vi "Execute.vi"(6 "QD Text":string, 7 "QD Plugins Dir":path, 8 "error in (no error)":errorcluster, 9 "Shift?":bool, 10 "Focus":enum8{"FP", "BD"}(ring), 11 "VI Refnum":refnum<vi>) -> (0 "error out":errorcluster)   [LabVIEW 2019, in "Script.lvlib"]
doc: "Executes scripts shortcuts defined in the Quick Drop arguments.\n\nHelp: Ctrl-Space + \"?\" + Ctrl-S\n\nCreated by: Ryan Pacini"
uses:
  Script.lvlib
  Definitions.ctl
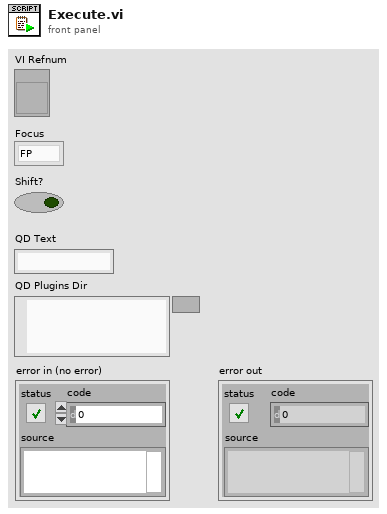
[diagram p1: front panel]
types:
  T1 = typedef "Script.lvlib/Definitions.ctl" = cluster{"plugins":cluster{"vi":path, "desc":string}[], "defaults":cluster{"uid":string, "name":string}[], "shortcuts":cluster{"shortcut":string, "uids":string[]}[], "defaults?":bool}
  T2 = enum16{"open", "replace", "create", "open or create", "replace or create", "replace or create with confirmation"}
  T3 = cluster{"name":string, "default":cluster{"uid":string, "name":string}}
  T4 = cluster{"name":string, "default":cluster{"uid":string, "name":string}}[]
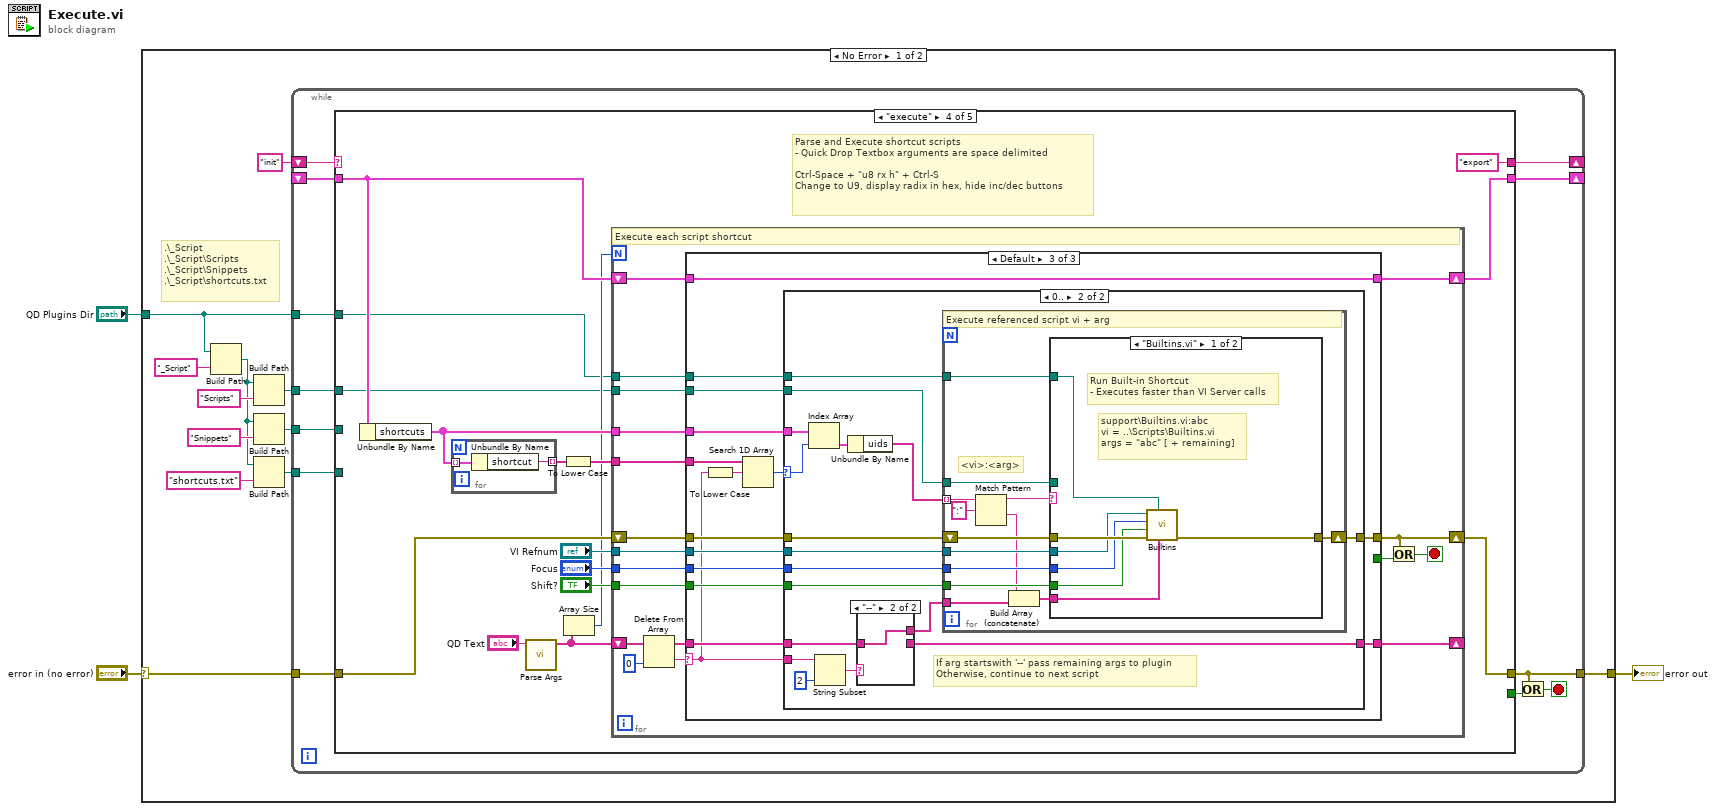
[diagram p0: block diagram]
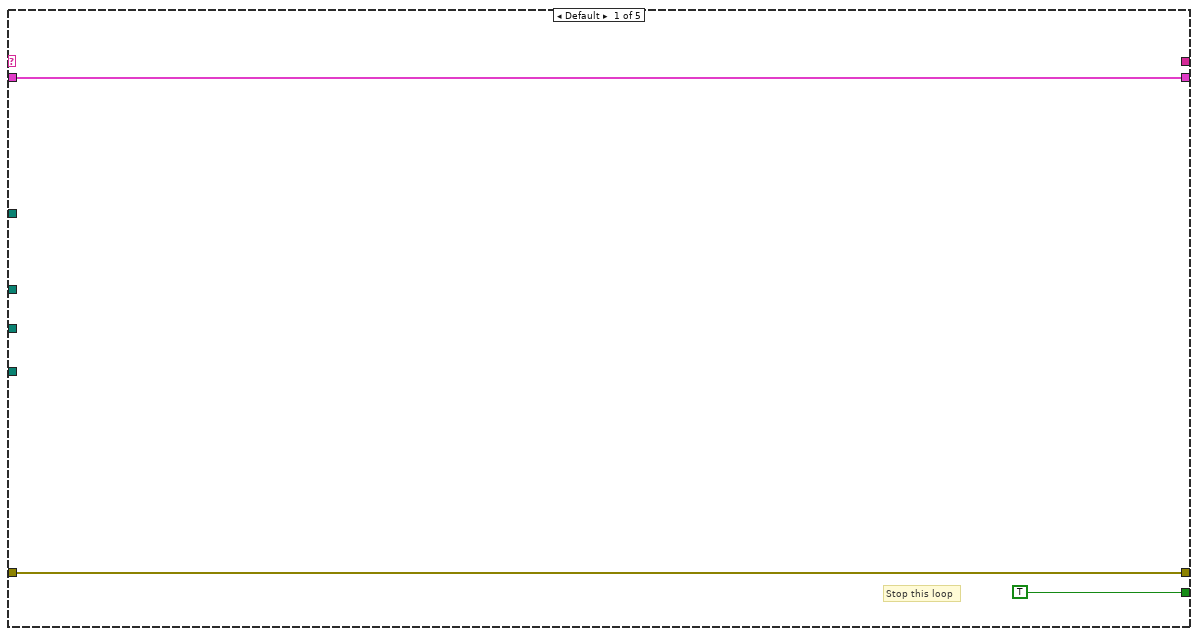
[diagram p2: hidden frame]
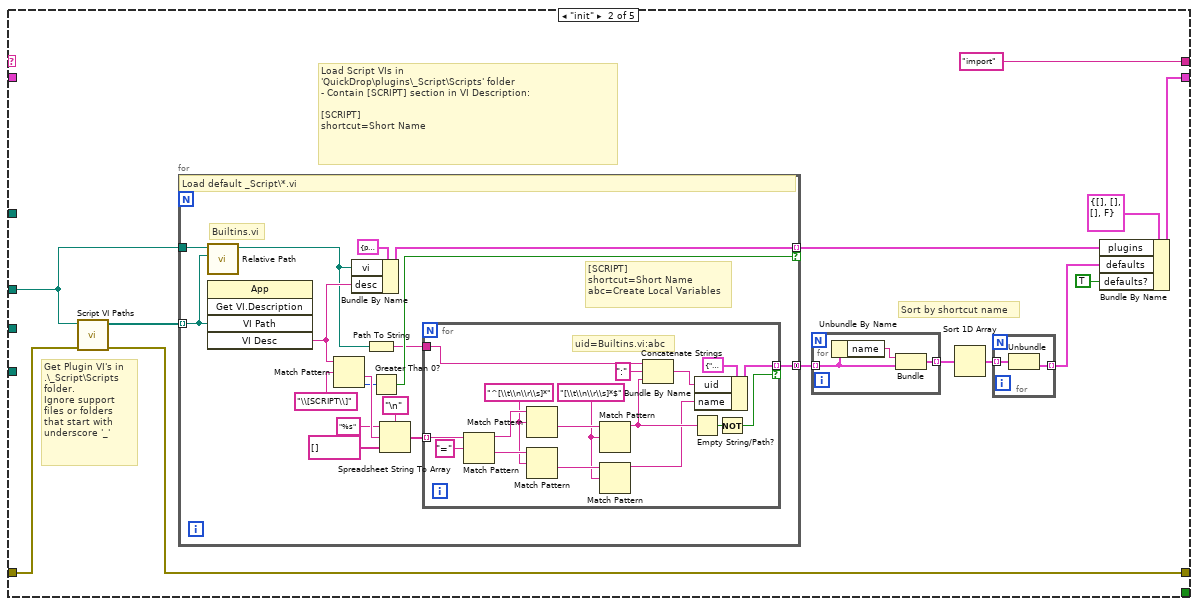
[diagram p3: hidden frame]
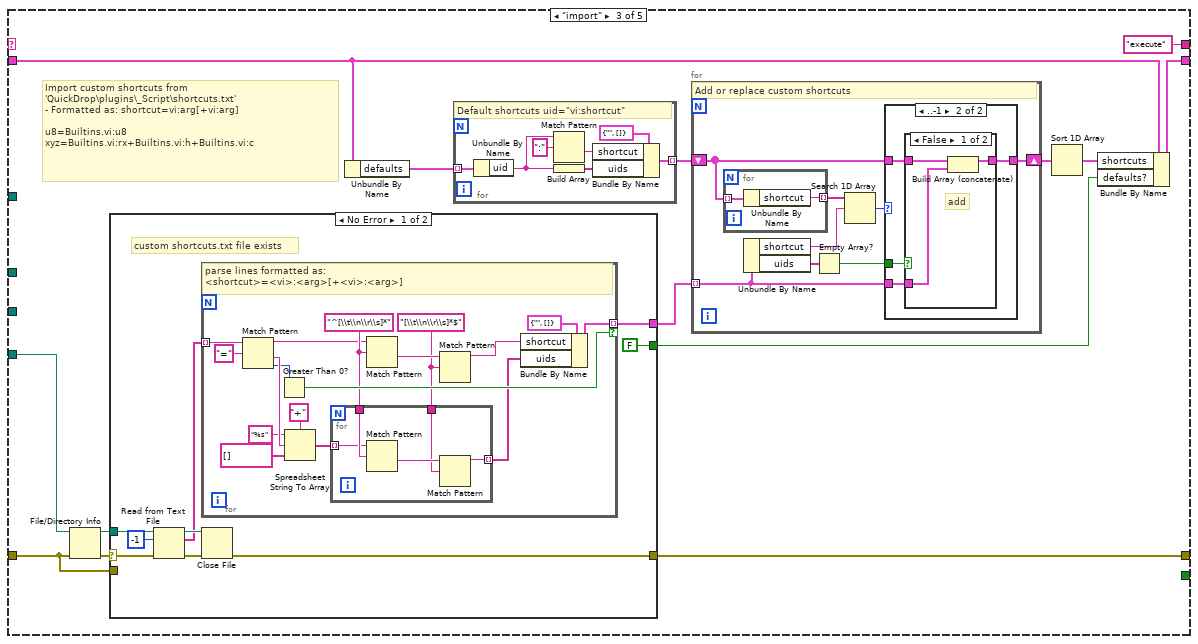
[diagram p4: hidden frame]
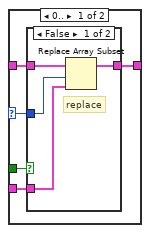
[diagram p5: hidden frame]
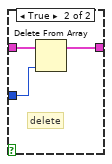
[diagram p6: hidden frame]
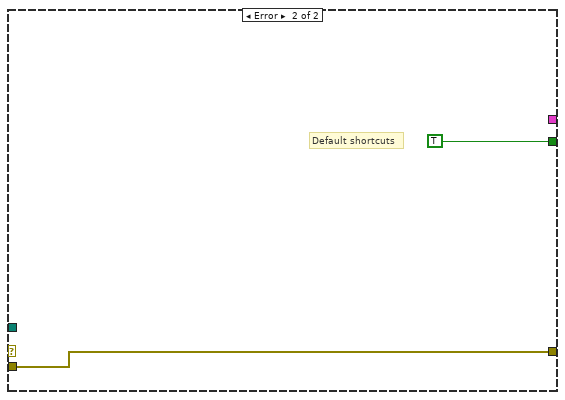
[diagram p8: hidden frame]
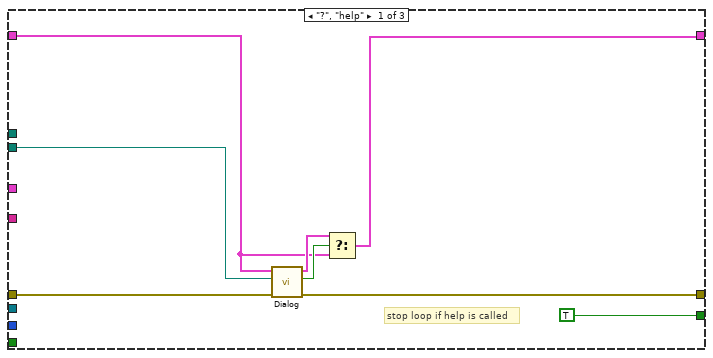
[diagram p9: hidden frame]
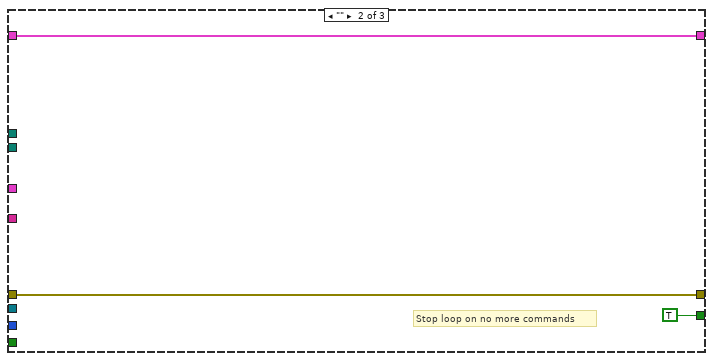
[diagram p10: hidden frame]
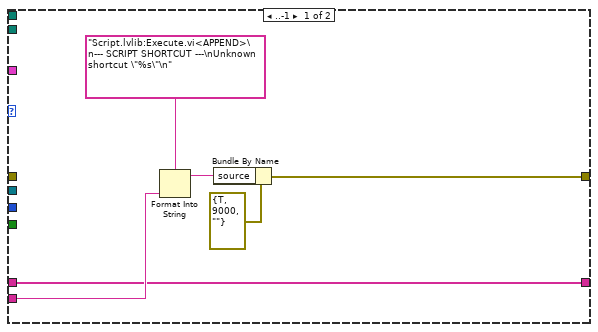
[diagram p11: hidden frame]
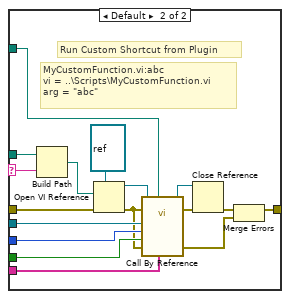
[diagram p13: hidden frame]
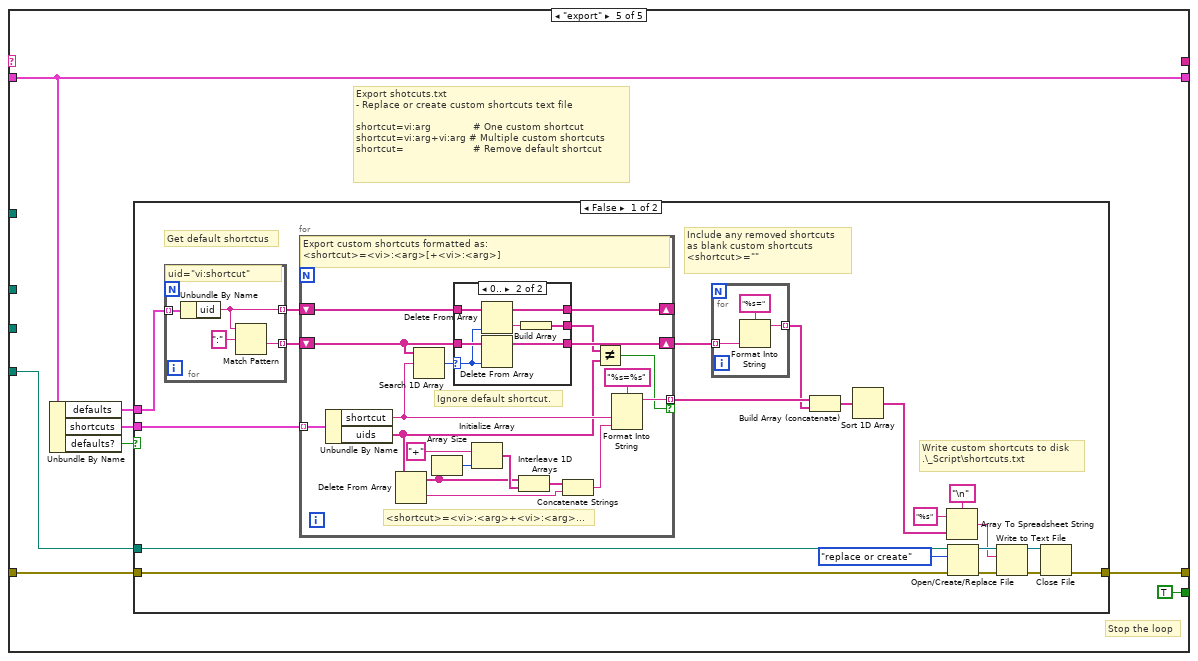
[diagram p14: hidden frame]
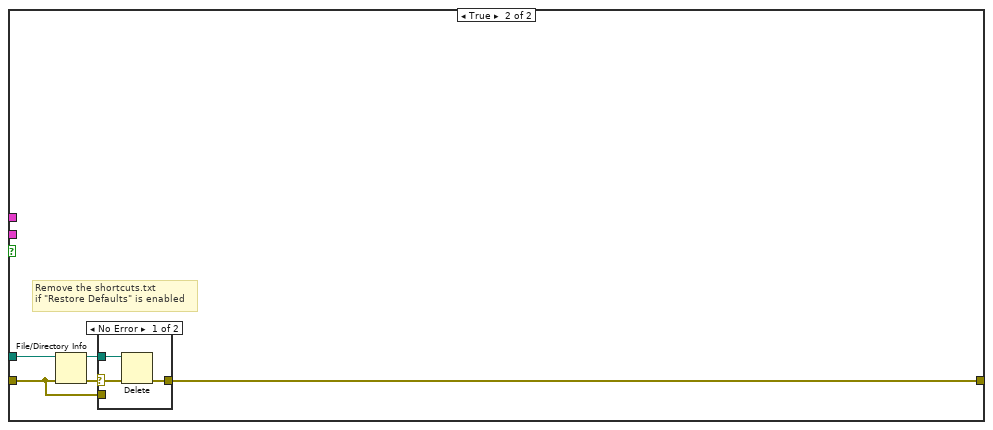
[diagram p16: hidden frame]
diagram:
  n1 = case shown="No Error" "error in (no error)" {
    selector: "error in (no error)" -> [w14 w362]
    tunnel: [w12 w362] -> w2
    tunnel: "QD Plugins Dir" -> [w10 _]
    frame No Error {
      # ".\\_Script\n.\\_Script\\Scripts\n.\\_Script\\Snippets\n.\\_Script\\shortcuts.txt"
      n2 = Build Path(base path=w10, name or relative path="_Script") -> (appended path=w4:path)
      n3 = Build Path(base path=w4, name or relative path="Scripts") -> (appended path=w8:path)
      n4 = Build Path(base path=w4, name or relative path="Snippets") -> (appended path=w5:path)
      n5 = Build Path(base path=w4, name or relative path="shortcuts.txt") -> (appended path=w9:path)
      n6 = while {
        tunnel: w14 -> [w27]
        shift-right: [w25] -> _
        shift-left: "init" -> [w26]
        shift-right: [w24] -> _
        shift-left: _ -> [w23]
        tunnel: [w22] -> w12
        tunnel: w10 -> [w19]
        tunnel: w9 -> [w18]
        tunnel: w8 -> [w17]
        tunnel: w5 -> [w16]
        stop <- w21 stop-if-true
        n7 = case shown="\"execute\"" w26 {
          tunnel: w27 -> [w29 w35 w92 w181 w297]
          tunnel: [_ "import" "execute" "export" _] -> w25
          tunnel: [w30 w42 w90 w175 w294] -> w24
          tunnel: w23 -> [w30 _ w86 w171 w294]
          tunnel: [w29 w34 w95 w177 w296] -> w22
          tunnel: [TRUE _ _ _ TRUE] -> w20
          tunnel: w19 -> [_ _ _ w166 _]
          tunnel: w18 -> [_ _ w91 _ w295]
          tunnel: w17 -> [_ w31 _ w167 _]
          tunnel: w16 -> [_ _ _ _ _]
          frame Default {
            # "Stop this loop"
          }
          frame "init" {
            # "Load Script VIs in \n'QuickDrop\\plugins\\_Script\\Scripts' folder\n- Contain [SCRIPT] section in VI Description:\n\n[SCRIPT]\nshortcut=Short Name"
            # "Get Plugin VI's in \n.\\_Script\\Scripts \nfolder.\nIgnore support \nfiles or folders\nthat start with\nunderscore '_'"
            # "Sort by shortcut name"
            n8 = call "Script VI Paths.vi"("error in (no error)"=w35, "Directory"=w31) -> ("error out"=w34:errorcluster, "VI Paths"=w33:path[])  [unwired: 8 in]
            n9 = for {
              tunnel: w33 -> [w64] mode=indexing
              tunnel: [w63] -> w40 mode=indexing if=w62
              tunnel: w31 -> [w61]
              tunnel: [w60] -> w39 mode=concatenating
              # "Builtins.vi"
              # "[SCRIPT]\nshortcut=Short Name\nabc=Create Local Variables"
              # "Load default _Script\\*.vi"
              n10 = call "Relative Path.vi"("Child"=w64, "Parent"=w61) -> ("Child Relative Path"=w49:path)  [unwired: 9 in]
              n11 = invoke class="App" method="Get VI.Description"("VI Path"=w64) -> ("VI Desc"=w51:string)  [unwired: 4 in, 4 out]
              n12 = Match Pattern(string=w51, regular expression="\\[SCRIPT\\]") -> (after substring=w58:string, offset past match=w53:i32)  [unwired: 1 in, 2 out]
              n13 = Bundle By Name(cluster=cluster{"vi":path, "desc":string} {"vi"=path "", "desc"=""} ("plugin"), "vi"=w49, "desc"=w51) -> (w63:cluster{"vi":path, "desc":string})
              n14 = Path To String(path=w49) -> (string=w50:string)
              n15 = Greater Than 0?(x=w53) -> (x > 0?=w62:bool)
              n16 = Spreadsheet String To Array(delimiter (Tab)="\n", format string="%s", spreadsheet string=w58, array type (2D Dbl)=string[] []) -> (array=w54:string[])
              n17 = for {
                tunnel: w54 -> [w81] mode=indexing
                tunnel: [w66] -> w60 mode=indexing if=w72
                tunnel: w50 -> [w70]
                w74 = "[\\t\\n\\r\\s]*$" ("regular expression")
                w75 = "^[\\t\\n\\r\\s]*" ("regular expression")
                # "uid=Builtins.vi:abc"
                n18 = Match Pattern(string=w81, regular expression="=") -> (before substring=w78:string, after substring=w76:string)  [unwired: 1 in, 2 out]
                n19 = Match Pattern(string=w78, regular expression=w75) -> (after substring=w79:string)  [unwired: 1 in, 3 out]
                n20 = Match Pattern(string=w76, regular expression=w75) -> (after substring=w77:string)  [unwired: 1 in, 3 out]
                n21 = Match Pattern(string=w79, regular expression=w74) -> (before substring=w69:string)  [unwired: 1 in, 3 out]
                n22 = Match Pattern(string=w77, regular expression=w74) -> (before substring=w65:string)  [unwired: 1 in, 3 out]
                n23 = Concatenate Strings(w70, ":" ("string"), w69) -> (w67:string)
                n24 = Empty String/Path?(string/path=w69) -> (empty?=w73:bool)
                n25 = Bundle By Name(cluster=cluster{"uid":string, "name":string} {"uid"="", "name"=""} ("default"), "uid"=w67, "name"=w65) -> (w66:cluster{"uid":string, "name":string})
                n26 = Not(x=w73) -> (.not. x?=w72:bool)
              }
            }
            n27 = for {
              tunnel: w39 -> [w47] mode=indexing
              tunnel: [w46] -> w38 mode=indexing
              n28 = Unbundle By Name(w47) -> ("name"=w48:string)
              n29 = Bundle("name"=w48, "default"=w47) -> (w46:T3)  [unwired: 1 in]
            }
            n30 = Sort 1D Array(array=w38) -> (sorted array=w37:T4)
            n31 = for {
              tunnel: w37 -> [w45] mode=indexing
              tunnel: [w44] -> w36 mode=indexing
              n32 = Unbundle(w45) -> ("default"=w44:cluster{"uid":string, "name":string})  [unwired: 1 out]
            }
            n33 = Bundle By Name(cluster=T1 {"plugins"=[], "defaults"=[], "shortcuts"=[], "defaults?"=FALSE} ("data"), "plugins"=w40, "defaults"=w36, "defaults?"=TRUE) -> (w42:T1)
          }
          frame "import" {
            # "Import custom shortcuts from \n'QuickDrop\\plugins\\_Script\\shortcuts.txt'\n- Formatted as: shortcut=vi:arg[+vi:arg]\n\nu8=Builtins.vi:u8\nxyz=Builtins.vi:rx+Builtins.vi:h+Builtins.vi:c"
            n34 = File/Directory Info(path=w91, error in=w92) -> (path out=w94:path, error out=w93:errorcluster)  [unwired: 5 out]
            n35 = case shown="No Error" w93 {
              selector: w93 -> [w140 _]
              tunnel: [w136 w165] -> w95
              tunnel: w94 -> [w141 _]
              tunnel: w92 -> [_ w165]
              tunnel: [FALSE TRUE] -> w87
              tunnel: [w133 _] -> w82
              frame No Error {
                # "custom shortcuts.txt file exists"
                n36 = Read from Text File(file (use dialog)=w141, count=-1, error in=w140) -> (refnum out=w137:refnum<file>, text=w134:string[], error out=w138:errorcluster)  [unwired: 1 in, 1 out]
                n37 = for {
                  tunnel: w134 -> [w158] mode=indexing
                  tunnel: [w149] -> w133 mode=indexing if=w151
                  w146 = "[\\t\\n\\r\\s]*$" ("regular expression")
                  w147 = "^[\\t\\n\\r\\s]*" ("regular expression")
                  # "parse lines formatted as:\n<shortcut>=<vi>:<arg>[+<vi>:<arg>]"
                  n38 = Match Pattern(string=w158, regular expression="=") -> (before substring=w145:string, after substring=w156:string, offset past match=w152:i32)  [unwired: 1 in, 1 out]
                  n39 = Greater Than 0?(x=w152) -> (x > 0?=w151:bool)
                  n40 = Spreadsheet String To Array(delimiter (Tab)="+", format string="%s", spreadsheet string=w156, array type (2D Dbl)=string[] []) -> (array=w143:string[])
                  n41 = for {
                    tunnel: w147 -> [w162]
                    tunnel: w146 -> [w161]
                    tunnel: w143 -> [w160] mode=indexing
                    tunnel: [w159] -> w142 mode=indexing
                    n42 = Match Pattern(string=w160, regular expression=w162) -> (after substring=w163:string)  [unwired: 1 in, 3 out]
                    n43 = Match Pattern(string=w163, regular expression=w161) -> (before substring=w159:string)  [unwired: 1 in, 3 out]
                  }
                  n44 = Match Pattern(string=w145, regular expression=w147) -> (after substring=w148:string)  [unwired: 1 in, 3 out]
                  n45 = Match Pattern(string=w148, regular expression=w146) -> (before substring=w144:string)  [unwired: 1 in, 3 out]
                  n46 = Bundle By Name(cluster=cluster{"shortcut":string, "uids":string[]} {"shortcut"="", "uids"=[]} ("shortcut"), "shortcut"=w144, "uids"=w142) -> (w149:cluster{"shortcut":string, "uids":string[]})
                }
                n47 = Close File(refnum=w137, error in=w138) -> (error out=w136:errorcluster)  [unwired: 1 out]
              }
              frame Error {
                # "Default shortcuts"
              }
            }
            n48 = Unbundle By Name(w86) -> ("defaults"=w85:cluster{"uid":string, "name":string}[])
            n49 = for {
              tunnel: w85 -> [w131] mode=indexing
              tunnel: [w129] -> w84 mode=indexing
              # "Default shortcuts uid=\"vi:shortcut\""
              n50 = Unbundle By Name(w131) -> ("uid"=w128:string)
              n51 = Match Pattern(string=w128, regular expression=":") -> (after substring=w126:string)  [unwired: 1 in, 3 out]
              n52 = Build Array(w128) -> (w130:string[])
              n53 = Bundle By Name(cluster=cluster{"shortcut":string, "uids":string[]} {"shortcut"="", "uids"=[]} ("shortcut"), "shortcut"=w126, "uids"=w130) -> (w129:cluster{"shortcut":string, "uids":string[]})
            }
            n54 = for {
              shift-right: [w100] -> w83
              shift-left: w84 -> [w103]
              tunnel: w82 -> [w99] mode=indexing
              # "Add or replace custom shortcuts"
              n55 = for {
                tunnel: w103 -> [w125] mode=indexing
                tunnel: [w124] -> w102 mode=indexing
                n56 = Unbundle By Name(w125) -> ("shortcut"=w124:string)
              }
              n57 = Unbundle By Name(w99) -> ("shortcut"=w101:string, "uids"=w97:string[])
              n58 = Empty Array?(array=w97) -> (empty?=w96:bool)
              n59 = Search 1D Array(1D array=w102, element=w101) -> (index of element=w98:i32)  [unwired: 1 in]
              n60 = case shown="..-1" w98 {
                selector: w98 -> [w105 _]
                tunnel: w103 -> [w108 w119]
                tunnel: [w107 w118] -> w100
                tunnel: w99 -> [w106 w117]
                tunnel: w96 -> [w104 w116]
                frame 0.. {
                  n61 = case shown="False" w104 {
                    tunnel: w108 -> [w112 w115]
                    tunnel: [w111 w113] -> w107
                    tunnel: w106 -> [w110 _]
                    tunnel: w105 -> [w109 w114]
                    frame False {
                      # "replace"
                      n62 = Replace Array Subset(array=w112, new element=w110, index=w109) -> (w111:cluster{"shortcut":string, "uids":string[]}[])
                    }
                    frame True {
                      # "delete"
                      n63 = Delete From Array(array=w115, index=w114) -> (array with subset deleted=w113:cluster{"shortcut":string, "uids":string[]}[])  [unwired: 1 in, 1 out]
                    }
                  }
                }
                frame ..-1 {
                  n64 = case shown="False" w116 {
                    tunnel: w119 -> [w122 w123]
                    tunnel: [w121 w123] -> w118
                    tunnel: w117 -> [w120 _]
                    frame False {
                      # "add"
                      n65 = Build Array (concatenate)(w122, w120) -> (w121:cluster{"shortcut":string, "uids":string[]}[])
                    }
                    frame True {
                      # "do not add"
                    }
                  }
                }
              }
            }
            n66 = Sort 1D Array(array=w83) -> (sorted array=w88:cluster{"shortcut":string, "uids":string[]}[])
            n67 = Bundle By Name(cluster=w86, "shortcuts"=w88, "defaults?"=w87) -> (w90:T1)
          }
          frame "execute" {
            # "Parse and Execute shortcut scripts\n- Quick Drop Textbox arguments are space delimited\n\nCtrl-Space + \"u8 rx h\" + Ctrl-S\nChange to U9, display radix in hex, hide inc/dec buttons"
            n68 = Unbundle By Name(w171) -> ("shortcuts"=w172:cluster{"shortcut":string, "uids":string[]}[])
            n69 = for {
              tunnel: w172 -> [w289] mode=indexing
              tunnel: [w288] -> w174 mode=indexing
              n70 = Unbundle By Name(w289) -> ("shortcut"=w288:string)
            }
            n71 = call "Parse Args.vi"("QD Text"="QD Text") -> ("args"=w168:string[])  [unwired: 10 in]
            n72 = To Lower Case(string=w174) -> (all lower case string=w173:string[])
            n73 = Array Size(array=w168) -> (size(s)=w169:i32)
            n74 = for {
              N: w169 -> [_]
              tunnel: w173 -> [w199]
              tunnel: w172 -> [w198]
              tunnel: "VI Refnum" -> [w196]
              tunnel: "Focus" -> [w195]
              tunnel: "Shift?" -> [w194]
              shift-right: [w190] -> w177
              shift-left: w181 -> [w197]
              shift-right: [w193] -> w175
              shift-left: w171 -> [w192]
              tunnel: w167 -> [w191]
              shift-right: [w184] -> _
              shift-left: w168 -> [w188]
              tunnel: w166 -> [w182]
              stop <- w186 stop-if-true
              # "Execute each script shortcut"
              n75 = Delete From Array(array=w188, index=0) -> (deleted portion=w183:string, array with subset deleted=w185:string[])  [unwired: 1 in]
              n76 = case shown="Default" w183 {
                selector: w183 -> [_ _ w213]
                tunnel: w199 -> [_ _ w225]
                tunnel: w198 -> [_ _ w223]
                tunnel: w197 -> [w207 w209 w222]
                tunnel: w196 -> [_ _ w221]
                tunnel: w195 -> [_ _ w220]
                tunnel: w194 -> [_ _ w219]
                tunnel: [w206 w209 w218] -> w190
                tunnel: [w202 w210 w217] -> w193
                tunnel: w192 -> [w203 w210 w217]
                tunnel: w191 -> [w201 _ w216]
                tunnel: [TRUE TRUE _] -> w189
                tunnel: w185 -> [_ _ w215]
                tunnel: [_ _ w214] -> w184
                tunnel: w182 -> [_ _ w211]
                frame "?", "help" {
                  # "stop loop if help is called"
                  n77 = call "Dialog.vi"("error in (no error)"=w207, "Scripts Dir"=w201, "Definitions in"=w203) -> ("error out"=w206:errorcluster, "commit?"=w205:bool, "Definitions out"=w204:T1)  [unwired: 6 in]
                  n78 = Select(t=w204, s=w205, f=w203) -> (s? t:f=w202:T1)
                }
                frame "" {
                  # "Stop loop on no more commands"
                }
                frame Default {
                  n79 = To Lower Case(string=w213) -> (all lower case string=w212:string)
                  n80 = Search 1D Array(1D array=w225, element=w212) -> (index of element=w224:i32)  [unwired: 1 in]
                  n81 = case shown="0.." w224 {
                    selector: w224 -> [_ w248]
                    tunnel: w223 -> [_ w247]
                    tunnel: w222 -> [_ w244]
                    tunnel: w221 -> [_ w243]
                    tunnel: w220 -> [_ w242]
                    tunnel: w219 -> [_ w241]
                    tunnel: [w230 w240] -> w218
                    tunnel: w216 -> [_ w239]
                    tunnel: w213 -> [w229 w237]
                    tunnel: w215 -> [w226 w235]
                    tunnel: [w226 w234] -> w214
                    tunnel: w211 -> [_ w232]
                    frame ..-1 {
                      n82 = Format Into String(format string="Script.lvlib:Execute.vi<APPEND>\n--- SCRIPT SHORTCUT ---\nUnknown shortcut \"%s\"\n" ("source"), w229) -> (resulting string=w227:string)  [unwired: 2 in, 1 out]
                      n83 = Bundle By Name(cluster=errorcluster {"status"=TRUE, "code"=9000, "source"=""} ("error IO"), "source"=w227) -> (w230:errorcluster)
                    }
                    frame 0.. {
                      # "If arg startswith '--' pass remaining args to plugin\nOtherwise, continue to next script"
                      n84 = Index Array(array=w247, index=w248) -> (element=w246:cluster{"shortcut":string, "uids":string[]})
                      n85 = String Subset(string=w237, length (rest)=2 ("length (rest)")) -> (substring=w236:string)  [unwired: 1 in]
                      n86 = Unbundle By Name(w246) -> ("uids"=w245:string[])
                      n87 = case shown="\"--\"" w236 {
                        tunnel: w235 -> [w249 w250]
                        tunnel: [w249 _] -> w234
                        tunnel: [_ w250] -> w233
                        frame Default {
                        }
                        frame "--" {
                        }
                      }
                      n88 = for {
                        tunnel: w245 -> [w257] mode=indexing
                        tunnel: w243 -> [w262]
                        tunnel: w242 -> [w261]
                        tunnel: w241 -> [w260]
                        shift-right: [w259] -> w240
                        shift-left: w244 -> [w263]
                        tunnel: w239 -> [w254]
                        tunnel: w233 -> [w253]
                        tunnel: w232 -> [w251]
                        # "<vi>:<arg>"
                        # "Execute referenced script vi + arg"
                        n89 = Match Pattern(string=w257, regular expression=":") -> (before substring=w255:string, after substring=w258:string)  [unwired: 1 in, 2 out]
                        n90 = Build Array (concatenate)(w258, w253) -> (w252:string[])
                        n91 = case shown="\"Builtins.vi\"" w255 {
                          selector: w255 -> [_ w275]
                          tunnel: w263 -> [w270 w287]
                          tunnel: w262 -> [w269 w284]
                          tunnel: w261 -> [w268 w283]
                          tunnel: w260 -> [w267 w282]
                          tunnel: [w266 w277] -> w259
                          tunnel: w254 -> [_ w274]
                          tunnel: w252 -> [w265 w272]
                          tunnel: w251 -> [w264 w271]
                          frame "Builtins.vi" {
                            # "support\\Builtins.vi:abc\nvi = ..\\Scripts\\Builtins.vi\nargs = \"abc\" [ + remaining]"
                            # "Run Built-in Shortcut\n- Executes faster than VI Server calls"
                            n92 = call "Builtins.vi"("args"=w265, "QD Plugins Dir"=w264, "error in (no error)"=w270, "Shift?"=w267, "Focus"=w268, "VI Refnum"=w269) -> ("error out"=w266:errorcluster)  [unwired: 5 in]
                          }
                          frame Default {
                            # "Run Custom Shortcut from Plugin"
                            # "MyCustomFunction.vi:abc\nvi = ..\\Scripts\\MyCustomFunction.vi\narg = \"abc\""
                            n93 = Build Path(base path=w274, name or relative path=w275) -> (appended path=w273:path)
                            n94 = Open VI Reference(type specifier VI Refnum (for type only)=refnum<vi> refnum, vi path=w273, error in (no error)=w287) -> (vi reference=w285:refnum<vi>, error out=w281:errorcluster)  [unwired: 3 in]
                            n95 = call-by-ref "?"(reference=w285, error in=w281, "args"=w272, "QD Plugins Dir"=w271, 8:"error in (no error)"=w281, "Shift?"=w282, "Focus"=w283, "VI Refnum"=w284) -> (reference out=w279:refnum<vi>, error out=w280:errorcluster, 0:"error out"=w276:errorcluster)  [unwired: 5 in]
                            n96 = Close Reference(reference=w279, error in (no error)=w280) -> (error out=w278:errorcluster)
                            n97 = Merge Errors(w278, w276) -> (w277:errorcluster)
                          }
                        }
                      }
                    }
                  }
                }
              }
              n98 = Or(x=w190, y=w189) -> (x .or. y?=w186:bool)
            }
          }
          frame "export" {
            # "Export shotcuts.txt\n- Replace or create custom shortcuts text file\n\nshortcut=vi:arg              # One custom shortcut\nshortcut=vi:arg+vi:arg # Multiple custom shortcuts\nshortcut=                       # Remove default shortcut"
            # "Stop the loop"
            n99 = Unbundle By Name(w294) -> ("defaults"=w290:cluster{"uid":string, "name":string}[], "shortcuts"=w293:cluster{"shortcut":string, "uids":string[]}[], "defaults?"=w291:bool)
            n100 = case shown="False" w291 {
              tunnel: w297 -> [w317 w353]
              tunnel: [w307 w354] -> w296
              tunnel: w295 -> [w306 w357]
              tunnel: w293 -> [w305 _]
              tunnel: w290 -> [w304 _]
              frame False {
                # "Include any removed shortcuts\nas blank custom shortcuts\n<shortcut>=\"\""
                # "Get default shortctus"
                # "Write custom shortcuts to disk\n.\\_Script\\shortcuts.txt"
                n101 = for {
                  tunnel: w304 -> [w324] mode=indexing
                  tunnel: [w322] -> w303 mode=indexing
                  tunnel: [w321] -> w302 mode=indexing
                  # "uid=\"vi:shortcut\""
                  n102 = Unbundle By Name(w324) -> ("uid"=w321:string)
                  n103 = Match Pattern(string=w321, regular expression=":") -> (after substring=w322:string)  [unwired: 1 in, 3 out]
                }
                n104 = for {
                  tunnel: [w343] -> w316 mode=indexing if=w334
                  tunnel: w305 -> [w342] mode=indexing
                  shift-right: [w326] -> w301
                  shift-left: w303 -> [w328]
                  shift-right: [w327] -> _
                  shift-left: w302 -> [w329]
                  # "<shortcut>=<vi>:<arg>+<vi>:<arg>..."
                  # "Ignore default shortcut."
                  # "Export custom shortcuts formatted as:\n<shortcut>=<vi>:<arg>[+<vi>:<arg>]"
                  n105 = Unbundle By Name(w342) -> ("shortcut"=w336:string, "uids"=w331:string[])
                  n106 = Delete From Array(array=w331) -> (deleted portion=w333:string, array with subset deleted=w330:string[])  [unwired: 2 in]
                  n107 = Search 1D Array(1D array=w328, element=w336) -> (index of element=w335:i32)  [unwired: 1 in]
                  n108 = Array Size(array=w330) -> (size(s)=w339:i32)
                  n109 = case shown="0.." w335 {
                    selector: w335 -> [_ w350]
                    tunnel: w329 -> [w345 w352]
                    tunnel: [_ w346] -> w325
                    tunnel: w328 -> [w344 w351]
                    tunnel: [w345 w349] -> w327
                    tunnel: [w344 w348] -> w326
                    frame ..-1 {
                    }
                    frame 0.. {
                      n110 = Delete From Array(array=w352, index=w350) -> (deleted portion=w347:string, array with subset deleted=w349:string[])  [unwired: 1 in]
                      n111 = Delete From Array(array=w351, index=w350) -> (array with subset deleted=w348:string[])  [unwired: 1 in, 1 out]
                      n112 = Build Array(w347) -> (w346:string[])
                    }
                  }
                  n113 = Initialize Array("+" ("delimiter (Tab)"), w339) -> (w332:string[])
                  n114 = Interleave 1D Arrays(w330, w332) -> (w338:string[])
                  n115 = Concatenate Strings(w338, w333) -> (w337:string)
                  n116 = Not Equal?(x=w325, y=w331) -> (x != y?=w334:bool)
                  n117 = Format Into String(format string="%s=%s", w336, w337) -> (resulting string=w343:string)  [unwired: 2 in, 1 out]
                }
                n118 = for {
                  tunnel: w301 -> [w319] mode=indexing
                  tunnel: [w318] -> w299 mode=indexing
                  n119 = Format Into String(format string="%s=", w319) -> (resulting string=w318:string)  [unwired: 2 in, 1 out]
                }
                n120 = Build Array (concatenate)(w316, w299) -> (w300:string[])
                n121 = Sort 1D Array(array=w300) -> (sorted array=w298:string[])
                n122 = Array To Spreadsheet String(delimiter (Tab)="\n", array=w298, 3:"%s" ("format string")) -> (spreadsheet string=w308:string)
                n123 = Open/Create/Replace File(file path (use dialog)=w306, error in=w317, operation (0:open)=T2."replace or create") -> (refnum out=w314:refnum<file>, error out=w315:errorcluster)  [unwired: 3 in, 1 out]
                n124 = Write to Text File(file (use dialog)=w314, text=w308, error in=w315) -> (refnum out=w313:refnum<file>, error out=w312:errorcluster)  [unwired: 1 in, 1 out]
                n125 = Close File(refnum=w313, error in=w312) -> (error out=w307:errorcluster)  [unwired: 1 out]
              }
              frame True {
                # "Remove the shortcuts.txt\nif \"Restore Defaults\" is enabled"
                n126 = File/Directory Info(path=w357, error in=w353) -> (path out=w355:path, error out=w356:errorcluster)  [unwired: 5 out]
                n127 = case shown="No Error" w356 {
                  selector: w356 -> [w360 _]
                  tunnel: w355 -> [w359 _]
                  tunnel: [w358 w361] -> w354
                  tunnel: w353 -> [_ w361]
                  frame No Error {
                    n128 = Delete(path (use dialog)=w359, error in=w360) -> (error out=w358:errorcluster)  [unwired: 3 in, 2 out]
                  }
                  frame Error {
                  }
                }
              }
            }
          }
        }
        n129 = Or(x=w22, y=w20) -> (x .or. y?=w21:bool)
      }
    }
    frame Error {
    }
  }
  "error out" <- w2
